vi "ActOnChangeToTiming.vi"() -> ()   [LabVIEW 2013]
uses:
  Controls/ExperimentControlEnum.ctl
  Controls/ExperimentControlCluster.ctl
  Controls/TimingControl.ctl
  Controls/TimingControlArray.ctl
panel:
  in  "Ctl Refnum":refnum<vi>
  out "queue out":refnum<queue>
  out "Timing Array out":T1 {"Timing Sequence"."Dt" format="%_3p"; "Timing Sequence"."Time" format="%_3p"}
  in  "Timing Array":T1 {"Timing Sequence"."Dt" format="%_3p"; "Timing Sequence"."Time" format="%_3p"}
  in  "Position":cluster{"Card":dbl, "Channel":dbl}
  in  "queue in":refnum<queue>
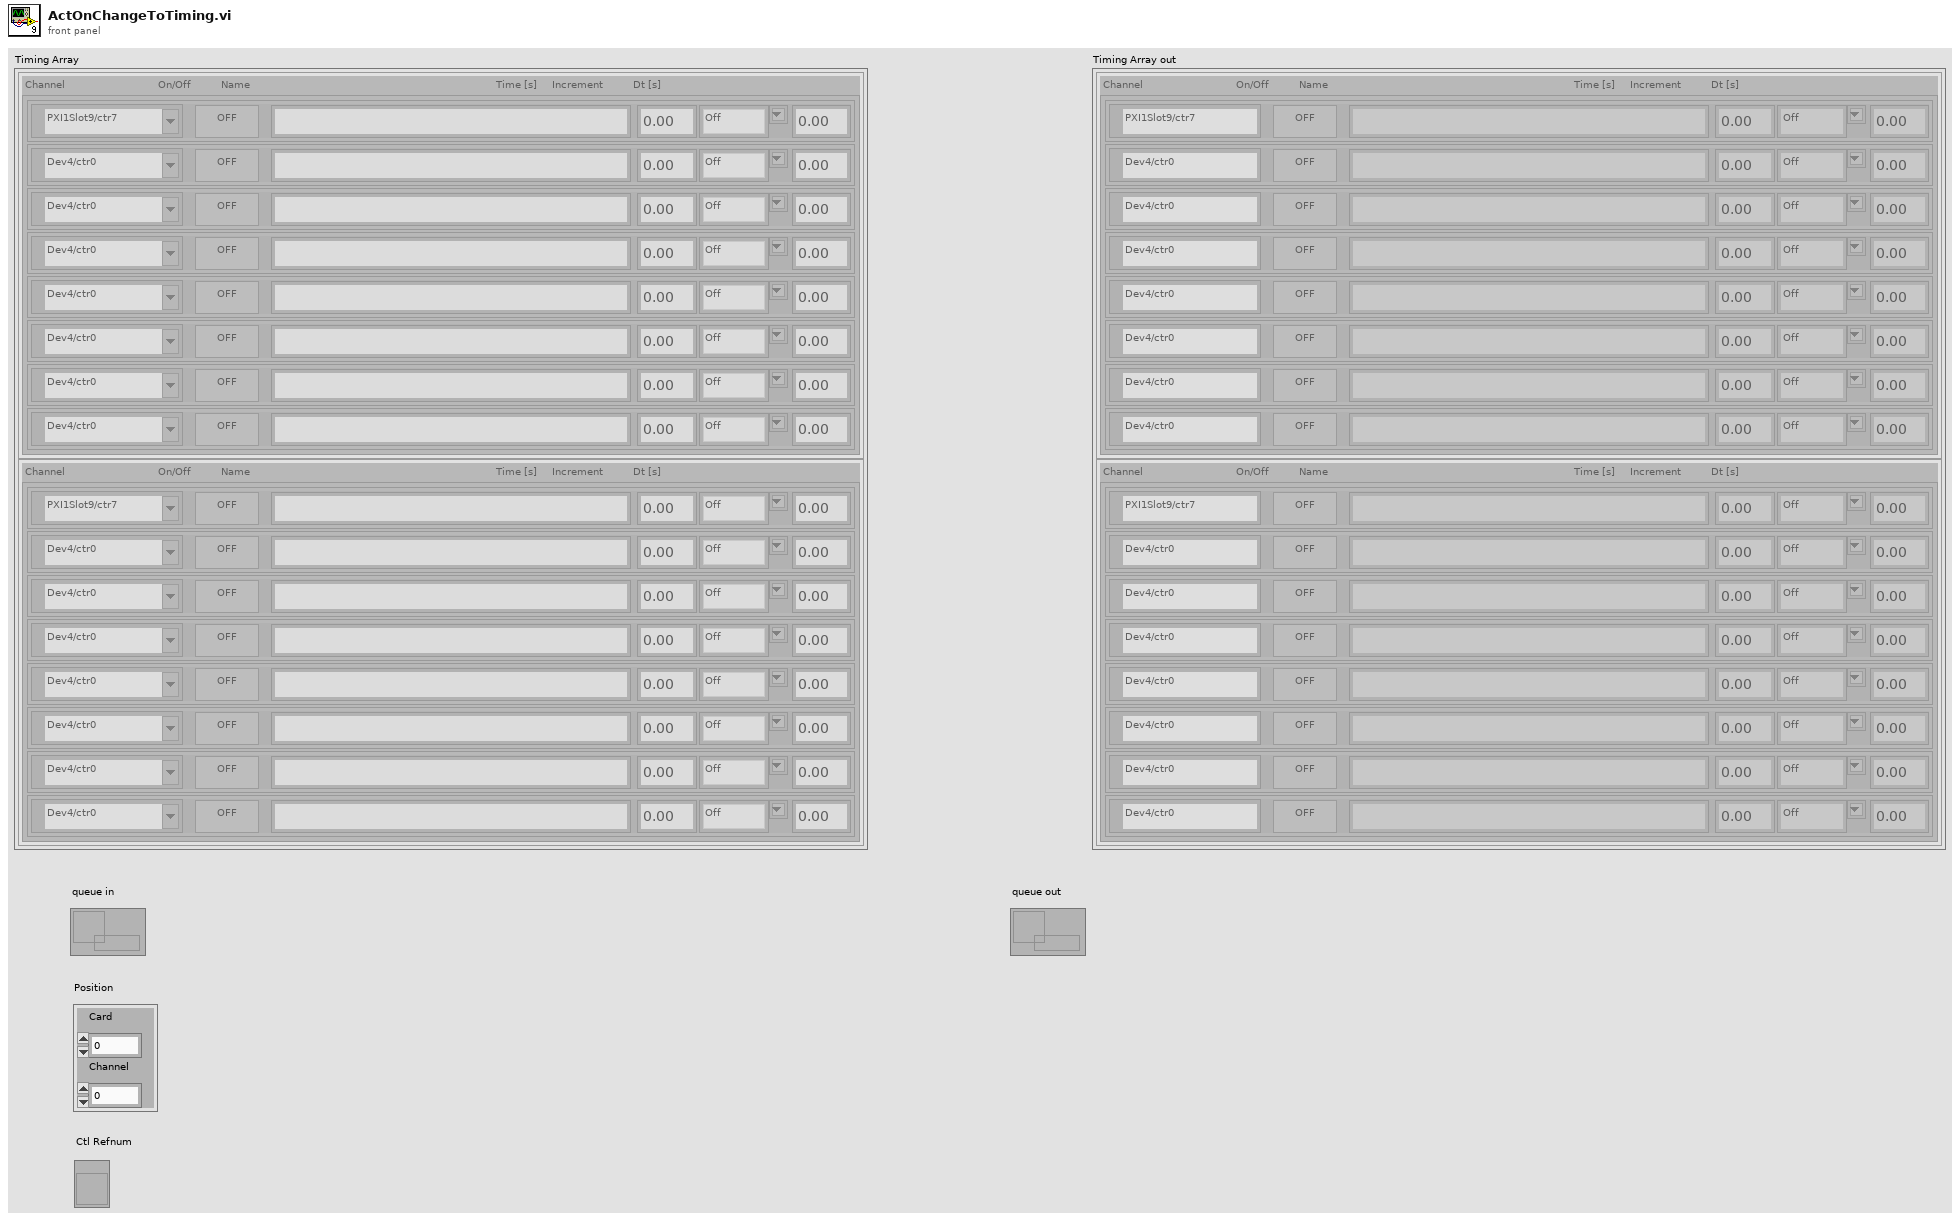
[diagram p1: front panel]
types:
  T1 = typedef "TimingControlArray.ctl" = T2[]
  T2 = typedef "TimingControl.ctl" = cluster{"Timing Sequence":cluster{"Active":bool, "counter":tag, "Channel Name":string, "Time":dbl, "Increment":string, "Dt":dbl}[]}
  T3 = typedef "ExperimentControlEnum.ctl" = enum16{"Idle", "Software Start", "Load Init", "Bank Charging", "Trigger Start", "Trigger In Progress", "Acquire PXI Data", "Turn Off DIO", "Shot Log Save", "Clean Up", "Auto Updated", "Stop VI", "Adjust Bounds", "Update Shot", "Config Load", "Print VI", "Config Save As", "Redraw Timing Plot", "Enable/Dis", "Increment Timing", "DIO Change"}
  T4 = cluster{"Active":bool, "counter":tag, "Channel Name":string, "Time":dbl, "Increment":string, "Dt":dbl}[]
  T5 = cluster{"Active":bool, "counter":tag, "Channel Name":string, "Time":dbl, "Increment":string, "Dt":dbl}
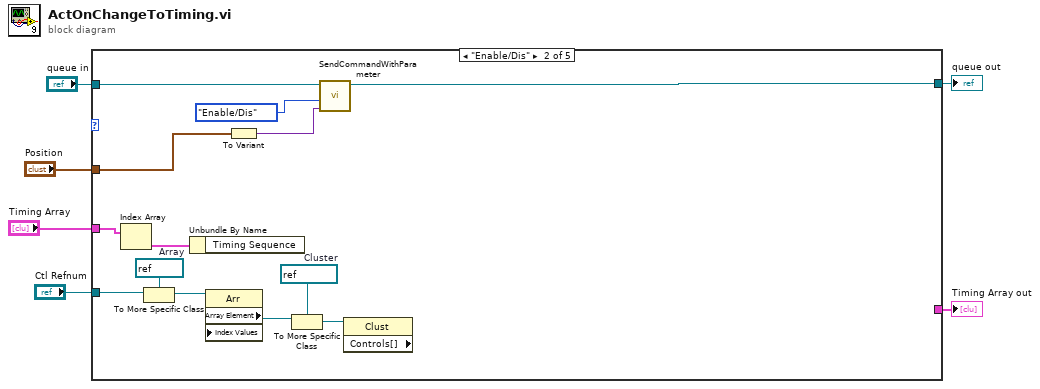
[diagram p0: block diagram]
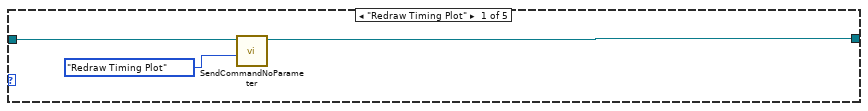
[diagram p2: hidden frame]
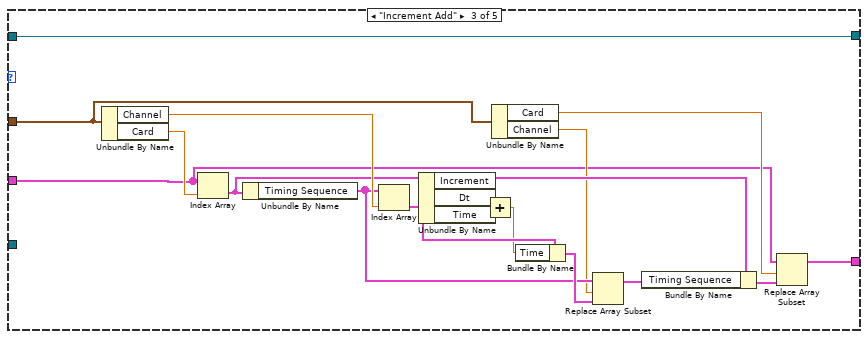
[diagram p3: hidden frame]
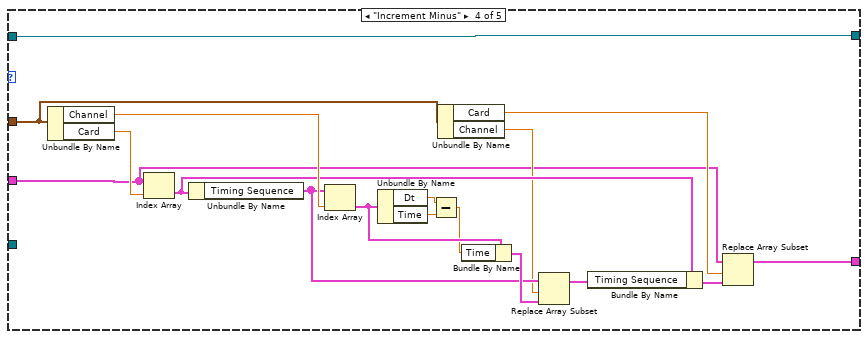
[diagram p4: hidden frame]
diagram:
  n1 = case shown="\"Enable/Dis\"" {
    selector: _ -> [_ _ _ _ _]
    tunnel: "Position" -> [_ w19 w27 w44 _]
    tunnel: "queue in" -> [w9 w22 w39 w56 w57]
    tunnel: [w8 w21 w39 w56 w57] -> w2
    tunnel: "Timing Array" -> [_ w11 w24 w40 _]
    tunnel: [_ _ w23 w41 _] -> w3
    tunnel: "Ctl Refnum" -> [_ w17 _ _ _]
    frame "Redraw Timing Plot" {
      n2 = call "SendCommandNoParameter.vi"("Command"=ExperimentControlEnum."Redraw Timing Plot" ("System State:  2"), "Command Q"=w9) -> ("Command Q"=w8:refnum<queue>)  [unwired: 9 in]
    }
    frame "Enable/Dis" {
      w13 = refnum<vi> refnum  # Cluster
      w16 = refnum<vi> refnum  # Array
      n3 = Index Array(array=w11) -> (element=w10:T2)  [unwired: 1 in]
      n4 = To More Specific Class(target class=w16, reference=w17) -> (specific class reference=w15:refnum<vi>)  [unwired: 1 in, 1 out]
      n5 = Unbundle By Name(w10) -> ()  [unwired: 1 out]
      n6 = property class="Arr" props=["Array Element", "Index Values"](reference=w15) -> ("Array Element"=w14:refnum<vi>)  [unwired: 2 in, 2 out]
      n7 = To Variant(anything=w19) -> (Variant=w18:variant)
      n8 = To More Specific Class(target class=w13, reference=w14) -> (specific class reference=w12:refnum<vi>)  [unwired: 1 in, 1 out]
      n9 = call "SendCommandWithParameter.vi"("Parameter"=w18, "Command"=ExperimentControlEnum."Enable/Dis" ("System State:  2"), "Command Q"=w22) -> ("Command Q"=w21:refnum<queue>)  [unwired: 8 in]
      n10 = property class="Clust" props=["Controls[]"](reference=w12) -> ()  [unwired: 1 in, 3 out]
    }
    frame "Increment Add" {
      n11 = Unbundle By Name(w27) -> ("Channel"=w34:dbl, "Card"=w28:dbl)
      n12 = Index Array(array=w24, index=w28) -> (element=w31:T2)
      n13 = Unbundle By Name(w31) -> ("Timing Sequence"=w32:T4)
      n14 = Index Array(array=w32, index=w34) -> (element=w36:T5)
      n15 = Unbundle By Name(w36) -> ("Dt"=w37:dbl, "Time"=w38:dbl)  [unwired: 1 out]
      n16 = Add(x=w37, y=w38) -> (x+y=w35:dbl)
      n17 = Unbundle By Name(w27) -> ("Card"=w25:dbl, "Channel"=w26:dbl)
      n18 = Bundle By Name(cluster=w36, "Time"=w35) -> (w33:T5)
      n19 = Replace Array Subset(array=w32, new element=w33, index=w26) -> (w30:T4)
      n20 = Bundle By Name(cluster=w31, "Timing Sequence"=w30) -> (w29:T2)
      n21 = Replace Array Subset(array=w24, new element=w29, index=w25) -> (w23:T1)
    }
    frame "Increment Minus" {
      n22 = Unbundle By Name(w44) -> ("Channel"=w51:dbl, "Card"=w45:dbl)
      n23 = Index Array(array=w40, index=w45) -> (element=w48:T2)
      n24 = Unbundle By Name(w48) -> ("Timing Sequence"=w49:T4)
      n25 = Index Array(array=w49, index=w51) -> (element=w53:T5)
      n26 = Unbundle By Name(w53) -> ("Dt"=w54:dbl, "Time"=w55:dbl)
      n27 = Subtract(x=w54, y=w55) -> (x-y=w52:dbl)
      n28 = Unbundle By Name(w44) -> ("Card"=w42:dbl, "Channel"=w43:dbl)
      n29 = Bundle By Name(cluster=w53, "Time"=w52) -> (w50:T5)
      n30 = Replace Array Subset(array=w49, new element=w50, index=w43) -> (w47:T4)
      n31 = Bundle By Name(cluster=w48, "Timing Sequence"=w47) -> (w46:T2)
      n32 = Replace Array Subset(array=w40, new element=w46, index=w42) -> (w41:T1)
    }
    frame "Do Nothing" {
    }
  }
  "Timing Array out" <- w3
  "queue out" <- w2
